vi "Execute.vi"(8 "error in (no error)":errorcluster, 10 "Abstract Consumer in":refnum<class "Abstract Consumer.lvclass">, 11 "Log Message in":refnum<class "Log Write Message.lvclass">) -> (0 "error out":errorcluster, 1 "Abstract Response out":refnum<class "Abstract Response Message.lvclass">, 2 "Abstract Consumer out":refnum<class "Abstract Consumer.lvclass">, 3 "Log Message out":refnum<class "Log Write Message.lvclass">, 4 "Stop?":bool)   [LabVIEW 2017, in "Messaging.lvlib" / "Log Write Message.lvclass"]
uses:
  Log Write Message.lvclass
  Consumer/Abstract Consumer/Abstract Consumer.lvclass
  Message/Abstract Response Message/Abstract Response Message.lvclass
  Abstract Log Consumer/Abstract Log Consumer.lvclass
  C:/git/ni/niveristand-custom-device-message-library/Source/Consumer/Abstract Consumer/Abstract Consumer.lvclass
  Log Write Message.lvclass/Log Write Message.ctl
  Read Values.vi
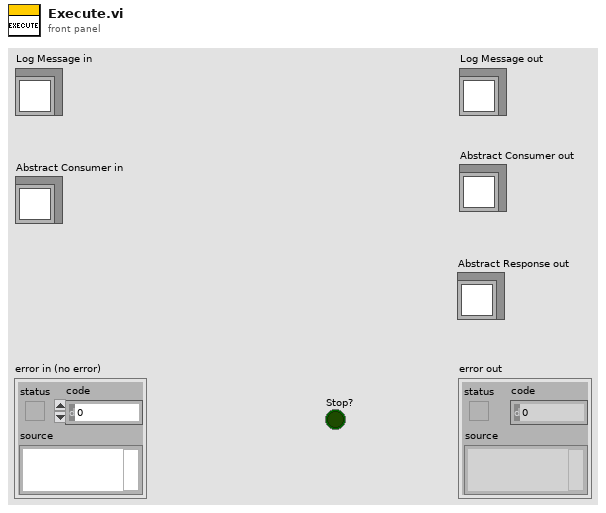
[diagram p1: front panel]
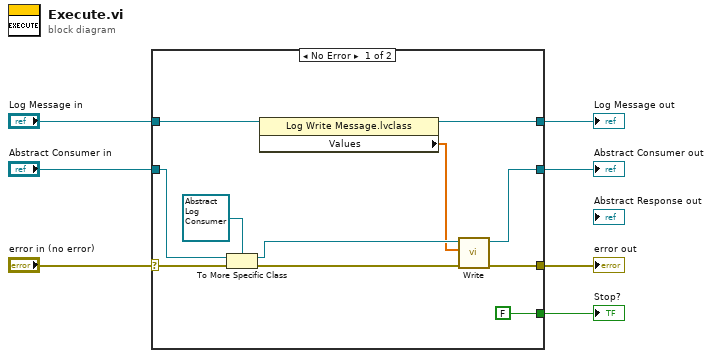
[diagram p0: block diagram]
diagram:
  n1 = case shown="No Error" "error in (no error)" {
    selector: "error in (no error)" -> [w17 w19]
    tunnel: "Abstract Consumer in" -> [w18 w20]
    tunnel: "Log Message in" -> [w11 w21]
    tunnel: [w13 w19] -> w4
    tunnel: [w10 w21] -> w3
    tunnel: [w12 w20] -> w2
    tunnel: [FALSE _] -> w1
    frame No Error {
      n2 = To More Specific Class(target class=refnum<class "Abstract Log Consumer.lvclass"> refnum ("Messaging.lvlib:Abstract Log Consumer.lvclass"), reference=w18, error in=w17) -> (specific class reference=w14:refnum<class "Abstract Log Consumer.lvclass">, error out=w15:errorcluster)
      n3 = property class="Log Write Message.lvclass"(reference=w11) -> (reference out=w10:refnum<class "Log Write Message.lvclass">, "Values"=w9:dbl[])  [unwired: 1 in, 1 out]
      n4 = call-dynamic "Write.vi"("error in (no error)"=w15, "Values"=w9, "Abstract Log Consumer in"=w14) -> ("error out"=w13:errorcluster, "Abstract Log Consumer out"=w12:refnum<class "Abstract Log Consumer.lvclass">)  [unwired: 7 in]
    }
    frame Error {
    }
  }
  "error out" <- w4
  "Log Message out" <- w3
  "Abstract Consumer out" <- w2
  "Stop?" <- w1
